vi "TrajectoryUtil_toPathWeaverJSON.vi"(7 "AlwaysOverWrite":bool, 8 "error in (no error)":errorcluster, 10 "inTRAJECTORY":T1 {"States"."POSE"."ROTATION"."SIN" format="%13.4f"; "States"."POSE"."ROTATION"."COS" format="%13.4f"; "States"."POSE"."ROTATION"."VALUE" format="%13.4f"; "States"."POSE"."TRANSLATION"."Y" format="%14.3f"; "States"."POSE"."TRANSLATION"."X" format="%14.3f"; "TotalTImeSecs" format="%20.3f"}, 11 "FileName":string="trajectory.json") -> (0 "error out":errorcluster, 4 "Full Filename":string)   [LabVIEW 2019, in "Trajectory_Library.lvlib"]
doc: "Exports a Trajectory to a PathWeaver-style JSON file.\n\nParameters:\n - Always Overwrite -- This optional terminal, if TRUE, will not prompt on WINDOWS to overwrite an existing file. On the RoboRIO the file is always overwritten. ( Default: False )\n - Trajectory - Trajectory data structure\n - FileName - File name string of the export json file\n - Error In - Error cluster (not used)\n\nReturns:\n - Error out - Returned error cluster"
uses:
  Trajectory_Library.lvlib
  TRAJECTORY.ctl
  TRAJ_STATE.ctl
  POSE2D.ctl
  TRANSLATION2D.ctl
  ROTATION2D.ctl
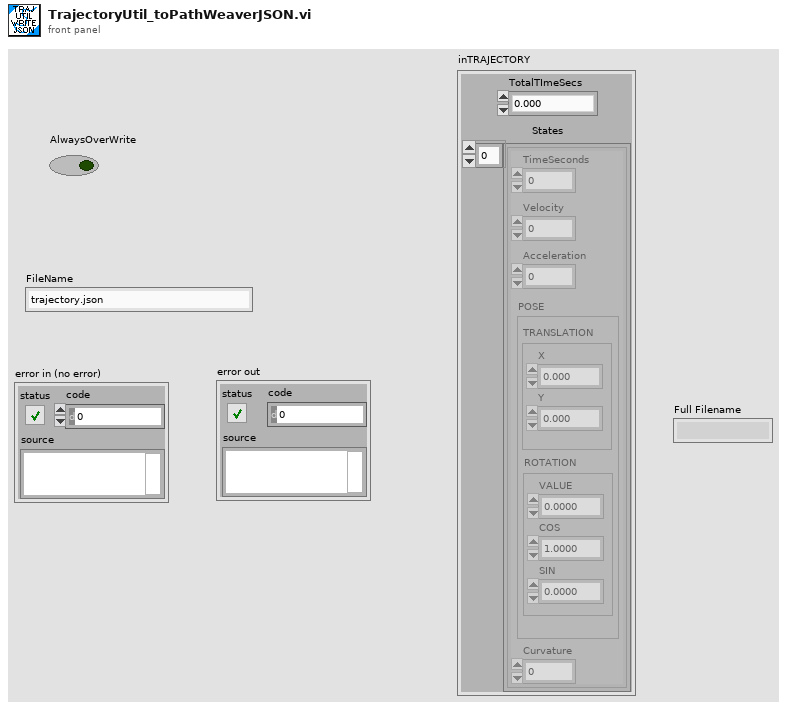
[diagram p1: front panel]
types:
  T1 = typedef "Trajectory_Library.lvlib/TRAJECTORY.ctl" = cluster{"TotalTImeSecs":dbl, "States":T2[]}
  T2 = typedef "Trajectory_Library.lvlib/TRAJ_STATE.ctl" = cluster{"TimeSeconds":dbl, "Velocity":dbl, "Acceleration":dbl, "POSE":T3, "Curvature":dbl}
  T3 = typedef "Trajectory_Library.lvlib/POSE2D.ctl" = cluster{"TRANSLATION":T4, "ROTATION":T5}
  T4 = typedef "Trajectory_Library.lvlib/TRANSLATION2D.ctl" = cluster{"X":dbl, "Y":dbl}
  T5 = typedef "Trajectory_Library.lvlib/ROTATION2D.ctl" = cluster{"VALUE":dbl, "COS":dbl, "SIN":dbl}
  T6 = enum16{"open", "replace", "create", "open or create", "replace or create", "replace or create with confirmation"}
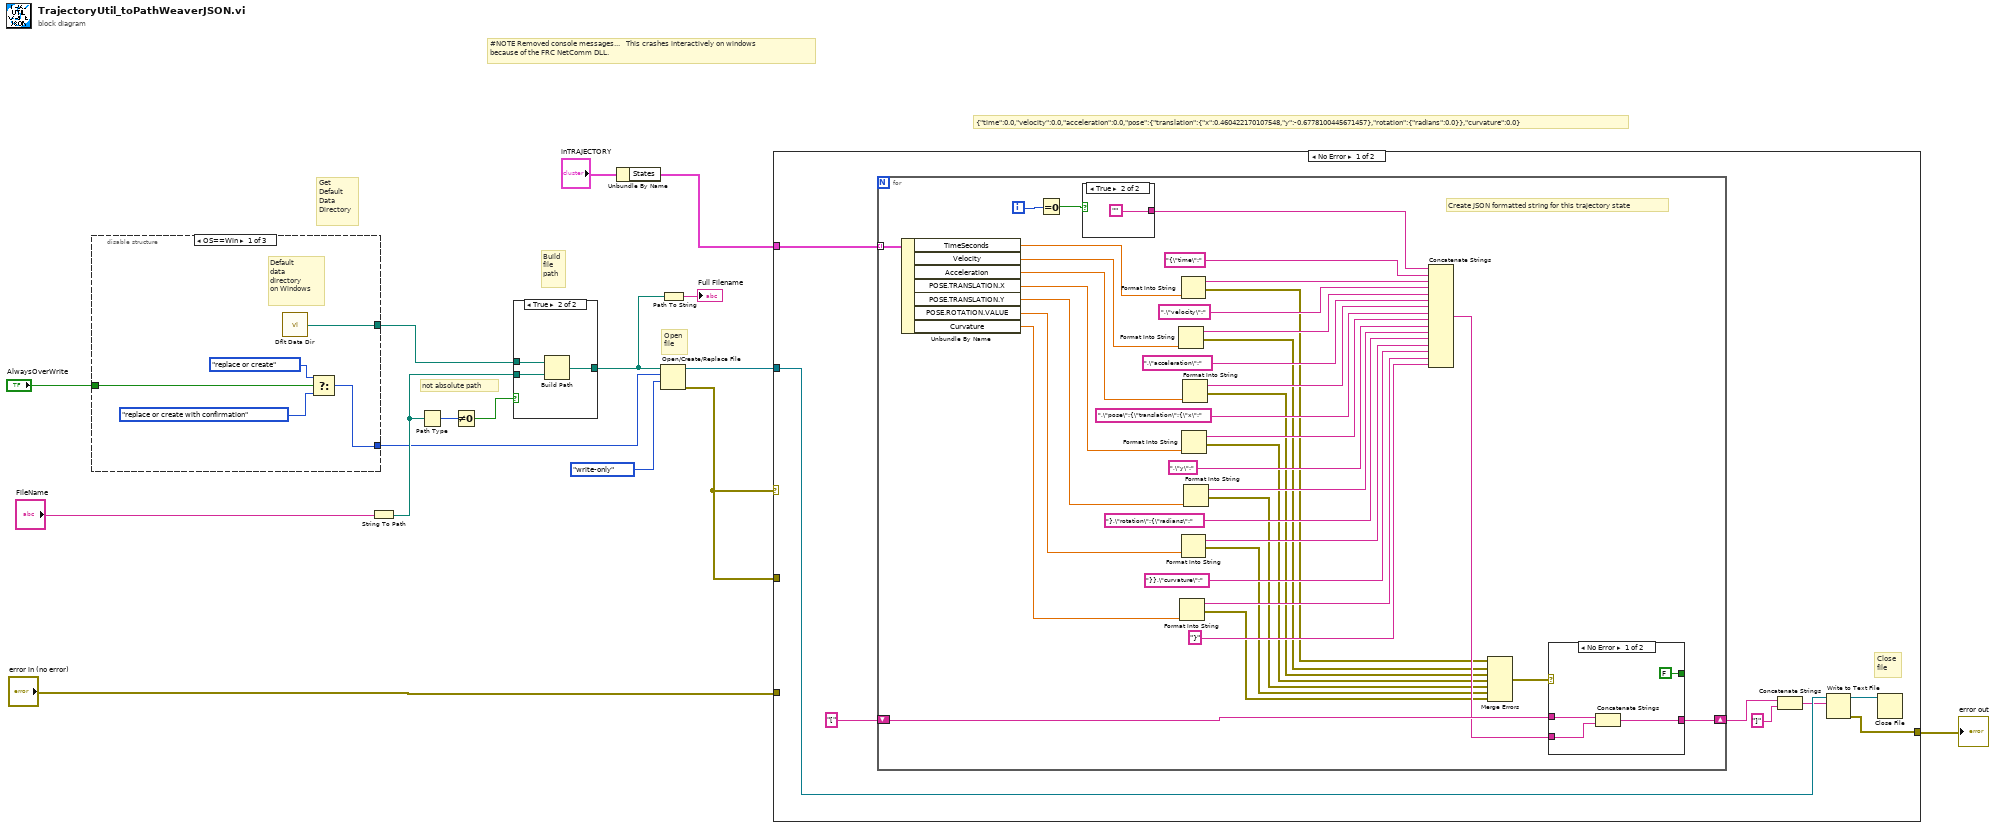
[diagram p0: block diagram]
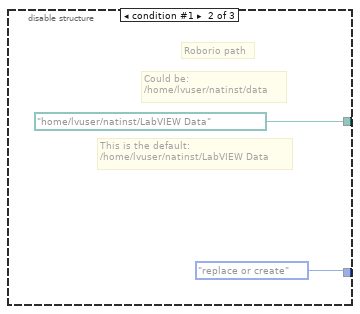
[diagram p3: hidden frame]
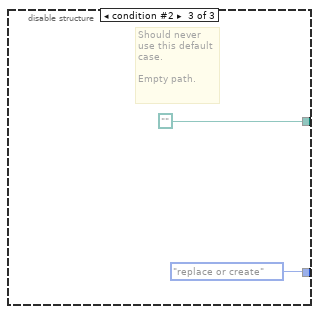
[diagram p4: hidden frame]
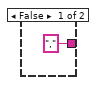
[diagram p5: hidden frame]
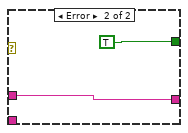
[diagram p6: hidden frame]
diagram:
  # "not absolute path"
  # "#NOTE Removed console messages...   This crashes interactively on windows \nbecause of the FRC NetComm DLL."
  # "{\"time\":0.0,\"velocity\":0.0,\"acceleration\":0.0,\"pose\":{\"translation\":{\"x\":0.460422170107548,\"y\":-0.6778100445671457},\"rotation\":{\"radians\":0.0}},\"curvature\":0.0}"
  # "Get\nDefault\nData\nDirectory"
  # "Open\nfile"
  # "Build\nfile\npath"
  n1 = disable-structure shown="OS==Win" {
    disable-tunnel: [w21 path "/home/lvuser/natinst/LabVIEW Data" path ""] -> w13
    disable-tunnel: [w17 T6."replace or create" ("operation (0:open)") T6."replace or create" ("operation (0:open)")] -> w4
    disable-tunnel: "AlwaysOverWrite" -> [w20 _ _]
    frame condition #0 (active) {
      # "Default\ndata\ndirectory\non Windows"
      n2 = call <vilib>:"Dflt Data Dir.vi"() -> ("App:Default Data Directory"=w21:path)
      n3 = Select(t=T6."replace or create" ("operation (0:open)"), s=w20, f=T6."replace or create with confirmation" ("operation (0:open)")) -> (s? t:f=w17:T6)
    }
    frame condition #1 {
      # "This is the default:\n/home/lvuser/natinst/LabVIEW Data"
      # "Could be:\n/home/lvuser/natinst/data"
      # "Roborio path"
    }
    frame condition #2 {
      # "Should never\nuse this default\ncase.\n\nEmpty path."
    }
  }
  n4 = String To Path(string="FileName") -> (path=w10:path)
  n5 = Path Type(1:w10) -> (0:w9:i16)
  n6 = Not Equal To 0?(x=w9) -> (x != 0?=w8:bool)
  n7 = case shown="True" w8 {
    tunnel: [w26 w29] -> w15
    tunnel: w13 -> [_ w28]
    tunnel: w10 -> [w26 w27]
    frame False {
    }
    frame True {
      n8 = Build Path(base path=w28, name or relative path=w27) -> (appended path=w29:path)
    }
  }
  n9 = Unbundle By Name("inTRAJECTORY") -> ("States"=w6:T2[])
  n10 = Open/Create/Replace File(file path (use dialog)=w15, operation (0:open)=w4, access (0:read/write)=enum16{"read/write", "read-only", "write-only"}."write-only") -> (refnum out=w5:refnum<file>, error out=w14:errorcluster)  [unwired: 3 in, 1 out]
  n11 = Path To String(path=w15) -> (string=→"Full Filename":string)
  n12 = case shown="No Error" w14 {
    tunnel: w14 -> [_ w83]
    tunnel: [w31 w83] -> w12
    tunnel: w6 -> [w37 _]
    tunnel: w5 -> [w33 _]
    tunnel: "error in (no error)" -> [_ _]
    frame No Error {
      # "Close\nfile"
      n13 = for {
        tunnel: w37 -> [w73] mode=indexing
        shift-right: [w46] -> w35
        shift-left: "[" -> [w47]
        i -> [w72]
        # "Create JSON formatted string for this trajectory state"
        n14 = Unbundle By Name(w73) -> ("TimeSeconds"=w54:dbl, "Velocity"=w53:dbl, "Acceleration"=w52:dbl, "POSE.TRANSLATION.X"=w51:dbl, "POSE.TRANSLATION.Y"=w50:dbl, "POSE.ROTATION.VALUE"=w49:dbl, "Curvature"=w48:dbl)
        n15 = Equal To 0?(x=w72) -> (x = 0?=w71:bool)
        n16 = case shown="True" w71 {
          tunnel: ["," ""] -> w70
          frame False {
          }
          frame True {
          }
        }
        n17 = Format Into String(w53) -> (resulting string=w66:string, error out=w43:errorcluster)  [unwired: 3 in]
        n18 = Format Into String(w48) -> (resulting string=w56:string, error out=w38:errorcluster)  [unwired: 3 in]
        n19 = Format Into String(w54) -> (resulting string=w68:string, error out=w44:errorcluster)  [unwired: 3 in]
        n20 = Format Into String(w49) -> (resulting string=w58:string, error out=w39:errorcluster)  [unwired: 3 in]
        n21 = Format Into String(w51) -> (resulting string=w62:string, error out=w41:errorcluster)  [unwired: 3 in]
        n22 = Format Into String(w52) -> (resulting string=w64:string, error out=w42:errorcluster)  [unwired: 3 in]
        n23 = Format Into String(w50) -> (resulting string=w60:string, error out=w40:errorcluster)  [unwired: 3 in]
        n24 = Concatenate Strings(w70, "{\"time\":", w68, ",\"velocity\":", w66, ",\"acceleration\":", w64, ",\"pose\":{\"translation\":{\"x\":", w62, ",\"y\":", w60, "},\"rotation\":{\"radians\":", w58, "}},\"curvature\":", w56, "}") -> (w45:string)
        n25 = Merge Errors(w44, w43, w42, w41, w40, w39, w38) -> (w74:errorcluster)
        n26 = case shown="No Error" w74 {
          tunnel: [FALSE TRUE] -> _
          tunnel: w47 -> [w79 w81]
          tunnel: [w78 w81] -> w46
          tunnel: w45 -> [w77 _]
          frame No Error {
            n27 = Concatenate Strings(w79, w77) -> (w78:string)
          }
          frame Error {
          }
        }
      }
      n28 = Concatenate Strings(w35, "]" ("string")) -> (w32:string)
      n29 = Write to Text File(file (use dialog)=w33, text=w32) -> (refnum out=w30:refnum<file>, error out=w31:errorcluster)  [unwired: 2 in, 1 out]
      n30 = Close File(refnum=w30) -> ()  [unwired: 1 in, 2 out]
    }
    frame Error {
      # "#NOTE Removed send error."
    }
  }
  "error out" <- w12
